vi "Processing Step.vi"(8 "error in (no error)":errorcluster, 11 "Complete Handler in":refnum<class "Complete Handler.lvclass">) -> (0 "error out":errorcluster, 2 "Step":T1[](array[typedef]), 3 "Complete Handler out":refnum<class "Complete Handler.lvclass">)   [LabVIEW 2020, in "HTTP Server.lvlib" / "Complete Handler.lvclass"]
uses:
  Complete Handler.lvclass
  Processing Step.ctl
  HTTP Server.lvlib
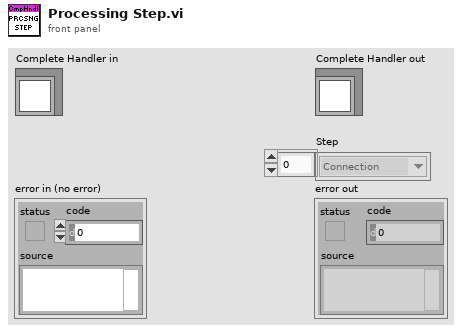
[diagram p1: front panel]
types:
  T1 = typedef "HTTP Server.lvlib/Processing Step.ctl" = enum16{"Connection", "Request", "Routing", "Controller Init", "Controller", "Response", "Cleanup", "Exception"}
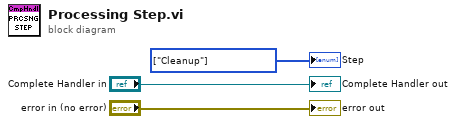
[diagram p0: block diagram]
diagram:
  w1 = T1[] [enum."Cleanup"] items=["Connection", "Request", "Routing", "Controller Init", "Controller", "Response", "Cleanup", "Exception"] ("Array")
  "error out" <- "error in (no error)"
  "Complete Handler out" <- "Complete Handler in"
  "Step" <- w1
